vi "Kinesis - KST101 - Move Relative.vi"() -> ()   [LabVIEW 2019]
doc: "Shows how to perform a relative motor move."
uses:
  C:/Program Files (x86)/National Instruments/LabVIEW 2019/user.lib/ThorKDC101/Kinesis_with_LabVIEW_Examples_LV12 - v3/Thorlabs.MotionControl.Controls.dll
  Thorlabs.MotionControl.Controls.dll
  C:/Program Files (x86)/National Instruments/LabVIEW 2019/user.lib/ThorKDC101/Kinesis_with_LabVIEW_Examples_LV12 - v3/Thorlabs.MotionControl.KCube.StepperMotorCLI.dll
  Thorlabs.MotionControl.KCube.StepperMotorCLI.dll
panel:
  in  "Step Size":dbl
  in  "Direction":i32(ring)=1 items=["Forward"=1, "Backward"=2]
  in  "?":bool
  in  "?":bool
  in  "?":bool
  in  "SerialNumber":string
  in  "KCubeStepperControl":refnum<k24>(container)
  # "Notes:"
  # "- Ensure that the appropriate .DLLs are copied into your Project Folder. Check that the correct bit type are used depending on your version of LabVIEW\ni.e. 32-bit or 64-bit.\n\n\n\n\n\n\n\n\n\n\n\n\n\n\n- Open the example VI through the LabVIEW Project Explorer to correctly load the User Interface from Thorlabs.MotionControl.Controls.dll."
  # "Thorlabs Hardware: KST101 - K-Cube Brushless DC Servo Motor Controller\n https://www.thorlabs.com/thorproduct.cfm?partnumber=KST101\n\nDescription: This VI will enable you to communicate with KST101 to control Stepper Motor Stages & Actuators. The VI will allow you to home the device and move it by any valid distance in any direction.\n\nInstructions: \n1) Connect your KST101 device to your PC & power the device, ensuring your stage/actutator is connected. For full device setup, the device product manual can be found on our website here. - https://www.thorlabs.com/thorproduct.cfm?partnumber=KST101\n2) Enter the device serial number below.\n3) Click 'Run' in the LabVIEW Toolbar.\n4) To end the Program click the 'STOP' button."
  # "Example Image of .NET Controller - VI opened via Project Explorer/ not opened via Project Explorer"
  # "VI Not Opened via Project Explorer"
  # "VI Opened via Project Explorer"
  # "- To explore the range of methods available, please visit the .NET API, included with your Kinesis software.\n\n- For tips on building your own VIs with Thorlabs Motion Control Hardware, please see our LabVIEW Guide here.\nhttps://www.thorlabs.com/newgrouppage9.cfm?objectgroup_id=10285"
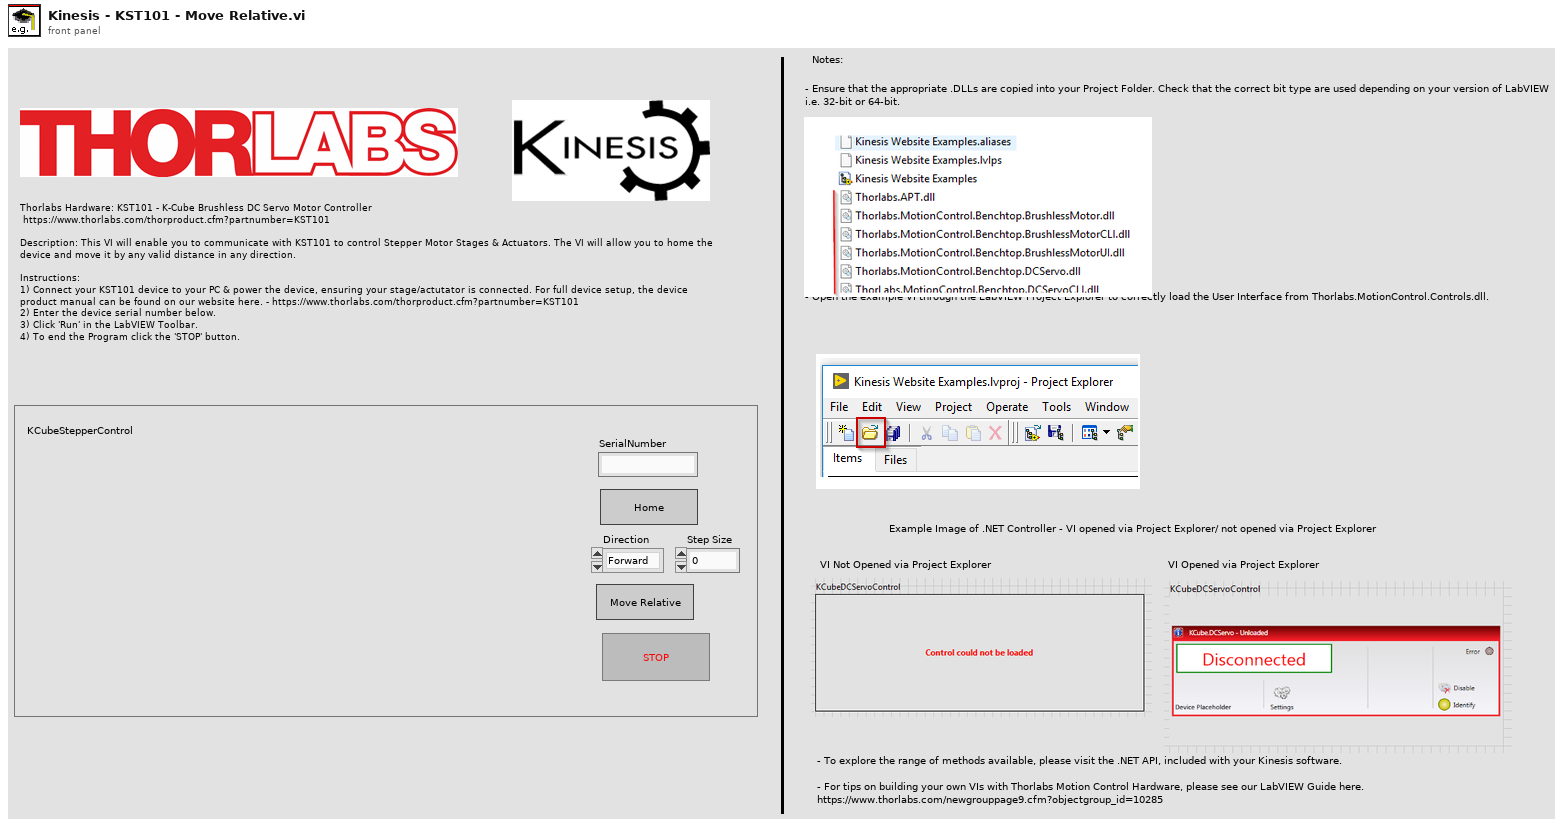
[diagram p1: front panel]
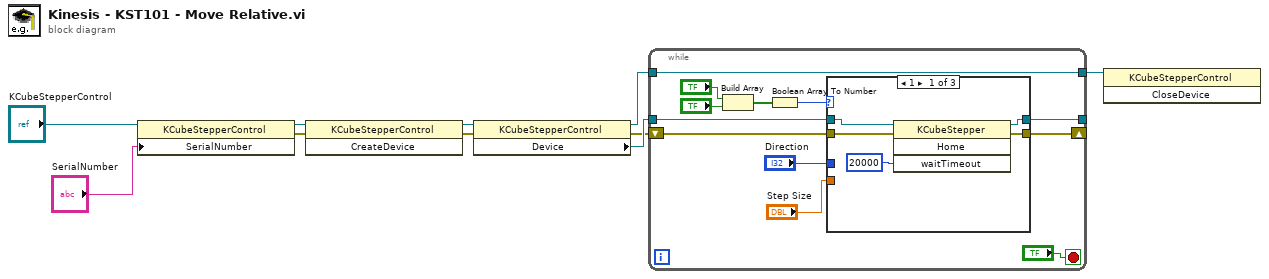
[diagram p0: block diagram]
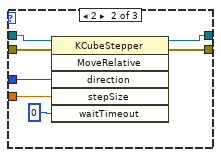
[diagram p2: hidden frame]
diagram:
  n1 = property class="KCubeStepperControl"(reference="KCubeStepperControl", "SerialNumber"="SerialNumber") -> (reference out=w8:refnum<k24>, error out=w5:errorcluster)  [unwired: 1 in]
  n2 = invoke class="KCubeStepperControl" method="CreateDevice"(reference=w8, error in=w5) -> (reference out=w7:refnum<k24>, error out=w4:errorcluster)  [unwired: 1 in, 1 out]
  n3 = property class="KCubeStepperControl"(reference=w7, error in=w4) -> (reference out=w1:refnum<k24>, error out=w3:errorcluster, "Device"=w6:refnum<k24>)
  n4 = while {
    tunnel: [w15] -> _
    shift-right: [w17] -> _
    shift-left: w3 -> [w16]
    tunnel: w6 -> [w14]
    tunnel: [w11] -> w2
    tunnel: w1 -> [w11]
    stop <- "?" stop-if-true
    n5 = Build Array("?", "?") -> (w19:bool[])
    n6 = Boolean Array To Number(Boolean array=w19) -> (number=w18:u32)
    n7 = case shown="1" w18 {
      tunnel: w14 -> [w27 w34 w35]
      tunnel: [w23 w28 w36] -> w17
      tunnel: w16 -> [w24 w29 w36]
      tunnel: [w25 w33 w35] -> w15
      tunnel: "Direction" -> [_ w32 _]
      tunnel: "Step Size" -> [_ w31 _]
      frame 1 {
        n8 = invoke class="KCubeStepper" method="Home"(reference=w27, error in=w24, "waitTimeout"=20000) -> (reference out=w25:refnum<k24>, error out=w23:errorcluster)  [unwired: 1 in, 2 out]
      }
      frame 2 {
        n9 = invoke class="KCubeStepper" method="MoveRelative"(reference=w34, error in=w29, "direction"=w32, "stepSize"=w31, "waitTimeout"=0) -> (reference out=w33:refnum<k24>, error out=w28:errorcluster)  [unwired: 1 in, 4 out]
      }
      frame Default {
      }
    }
  }
  n10 = invoke class="KCubeStepperControl" method="CloseDevice"(reference=w2) -> ()  [unwired: 2 in, 3 out]
